vi "ILABW_GetVI.vi"(4 "path":string) -> (0 "errorOut":string, 1 "name":string)   [LabVIEW 2012]
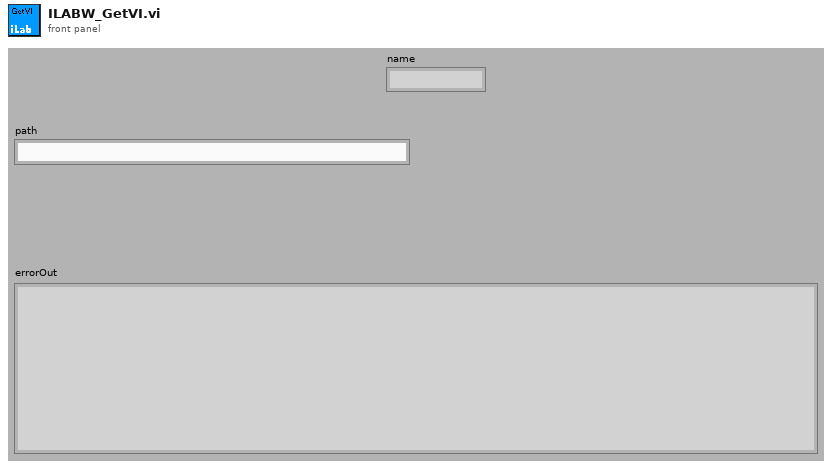
[diagram p1: front panel]
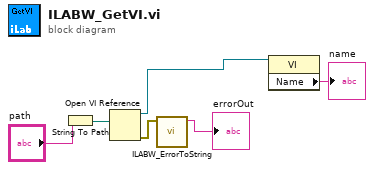
[diagram p0: block diagram]
diagram:
  n1 = String To Path(string="path") -> (path=w3:path)
  n2 = Open VI Reference(vi path=w3) -> (vi reference=w2:refnum<vi>, error out=w6:errorcluster)  [unwired: 5 in]
  n3 = call "ILABW_ErrorToString.vi"("errorIn"=w6) -> ("errorOut"=→"errorOut":string)  [unwired: 10 in]
  n4 = property class="VI"(reference=w2) -> ("Name"=→"name":string)  [unwired: 1 in, 2 out]
